vi "FA_WriteXML.vi"(6 "Error In":errorcluster, 7 "XML String":string, 8 "Special Type":T1) -> (0 "Error Out":errorcluster)   [LabVIEW 2014, in "FA_LocalStore.lvlib"]
doc: "Writes new XML to LocalStore for a given Special Type."
uses:
  FA_LocalStore.lvlib
  FA_LSSpecialTypes.ctl
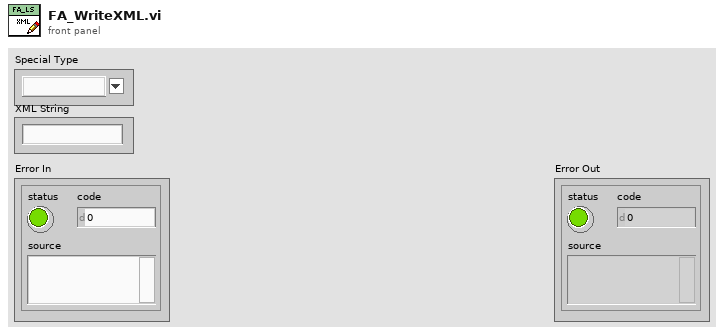
[diagram p1: front panel]
types:
  T1 = typedef "FA_LocalStore.lvlib/FA_LSSpecialTypes.ctl" = string
  T2 = typedef "FA_LocalStore.lvlib/FA_LSRef.ctl" = cluster{"eTag INI Refnum":T3, "XML Refnum Array":refnum<file>[]}
  T3 = typedef "NI_LVConfig.lvlib/Config Data RefNum.ctl" = refnum<k1>
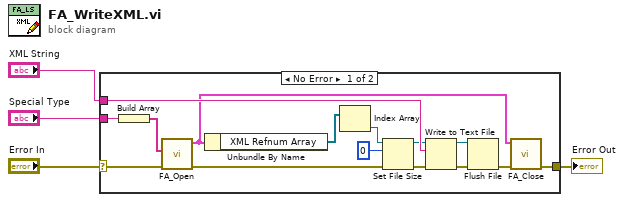
[diagram p0: block diagram]
diagram:
  n1 = case shown="No Error" "Error In" {
    selector: "Error In" -> [w6 w20]
    tunnel: [w7 w20] -> w3
    tunnel: "Special Type" -> [w10 _]
    tunnel: "XML String" -> [w19 _]
    frame No Error {
      n2 = Build Array(w10) -> (w9:T1[])
      n3 = call "FA_Open.vi"("Error In"=w6, "Special Types Array"=w9) -> ("Error Out"=w5:errorcluster, "FA_LS Ref"=w8:T2)  [unwired: 8 in]
      n4 = Unbundle By Name(w8) -> ("XML Refnum Array"=w18:refnum<file>[])
      n5 = Index Array(array=w18) -> (element=w17:refnum<file>)  [unwired: 1 in]
      n6 = Set File Size(4:w5, 6:i64 0 ("size (in bytes)"), 7:w17) -> (0:w15:errorcluster, 3:w16:refnum<file>)
      n7 = Write to Text File(file (use dialog)=w16, text=w19, error in=w15) -> (refnum out=w12:refnum<file>, error out=w13:errorcluster)  [unwired: 1 in, 1 out]
      n8 = Flush File(refnum=w12, error in=w13) -> (error out=w11:errorcluster)  [unwired: 1 out]
      n9 = call "FA_Close.vi"("Error In"=w11, "FA_LS Ref"=w8) -> ("Error Out"=w7:errorcluster)  [unwired: 9 in]
    }
    frame Error {
    }
  }
  "Error Out" <- w3
